vi "motor control 4.vi"(0 "Fine":u16, 1 "proportional gain (Kc)":dbl, 2 "Manual control":dbl, 3 "reinitialize? (F)":bool, 4 "derivative time (Td, min)":dbl, 5 "error in (no error)":errorcluster, 6 "integral time (Ti, min)":dbl, 7 "cycle\"i\"":i32, 8 "velocità desiderata":dbl, 9 "Stoppa ciclo":bool, 10 "offset":dbl, 11 "auto? (T)":bool=TRUE, 12 "delta t":u32) -> (14 "pwm out":dbl, 15 "Boolean":bool, 19 "error out":errorcluster)   [LabVIEW 2017]
uses:
  <vilib>/functionblocks/Control/PID/PID.vi
  <vilib>/functionblocks/FB Core/FB Core.xnode
  <vilib>/functionblocks/FB Property/FB Overlay DBL.ctl
  <vilib>/functionblocks/NI_FunctionBlock Libraries.lvlib
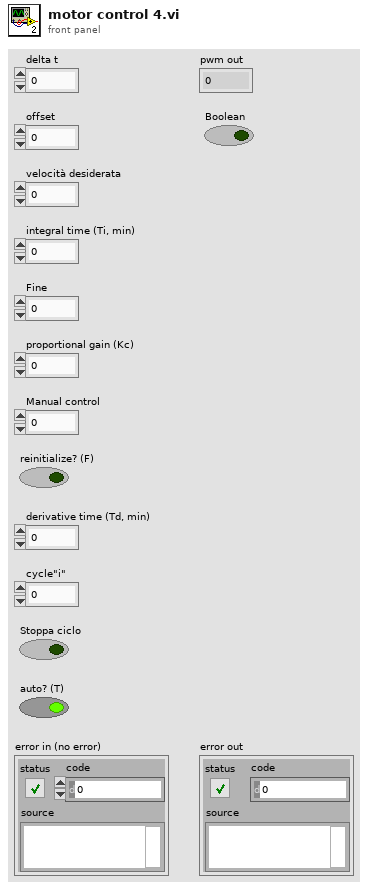
[diagram p1: front panel]
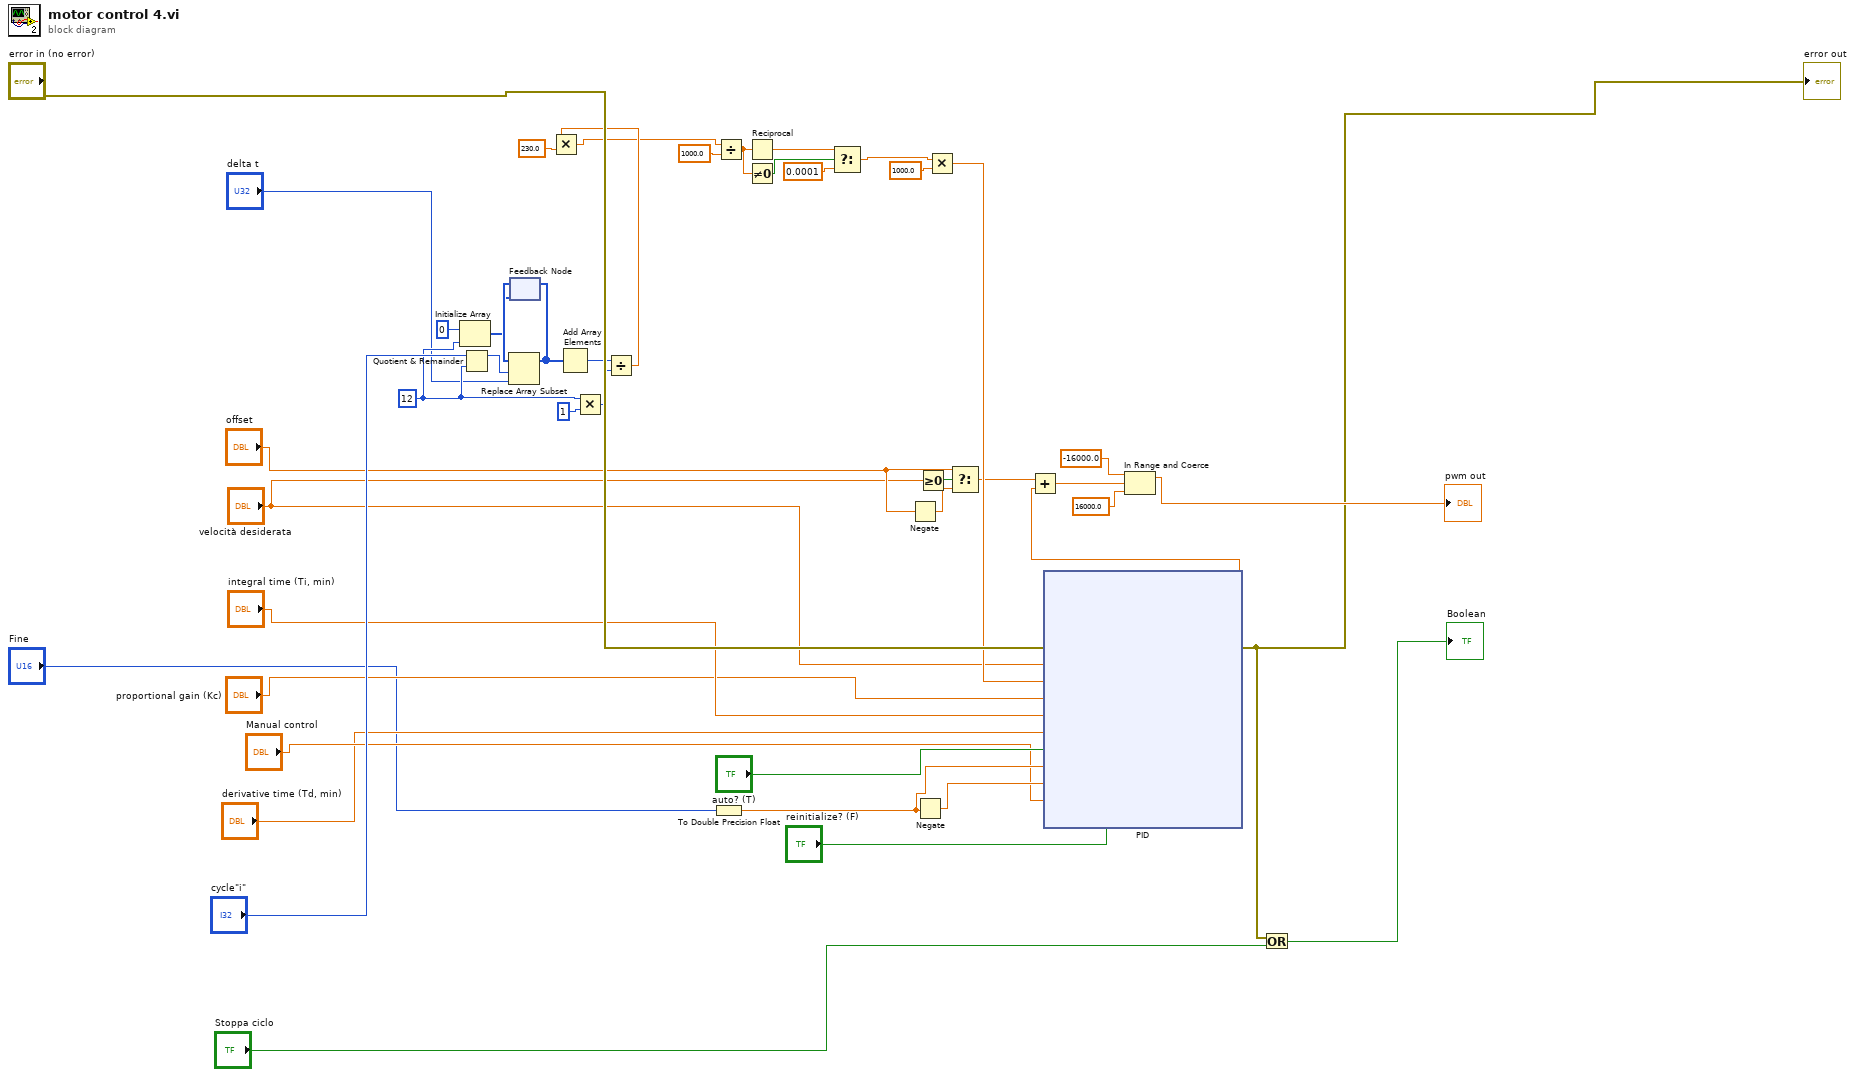
[diagram p0: block diagram]
diagram:
  w39 = 12 ("dimension size")
  n1 = Initialize Array(0, w39) -> (w40:i32[])
  n2 = Quotient & Remainder(x="cycle\"i\"", y=w39) -> (x-y*floor(x/y)=w32:i32)  [unwired: 1 out]
  n3 = feedback #1(w40) -> (w42:i32[])
  n4 = Replace Array Subset(array=w42, new element="delta t", index=w32) -> (w41:i32[])
  n5 = feedback-in #1(w41) -> ()
  n6 = Add Array Elements(numeric array=w41) -> (sum=w21:i32)
  n7 = Multiply(x=w39, y=1) -> (x*y=w34:i32)
  n8 = Divide(x=w21, y=w34) -> (x/y=w22:dbl)
  n9 = Multiply(x=w22, y=230.0) -> (x*y=w16:dbl)
  n10 = To Double Precision Float(number="Fine") -> (double precision float=w31:dbl)
  n11 = Divide(x=w16, y=1000.0) -> (x/y=w18:dbl)
  n12 = Reciprocal(x=w18) -> (1/x=w12:dbl)
  n13 = Not Equal To 0?(x=w18) -> (x != 0?=w13:bool)
  n14 = Select(t=w12, s=w13, f=0.0001) -> (s? t:f=w19:dbl)
  n15 = Negate(x="offset") -> (-x=w24:dbl)
  n16 = Negate(x=w31) -> (-x=w30:dbl)
  n17 = Greater Or Equal To 0?(x="velocità desiderata") -> (x >= 0?=w25:bool)
  n18 = Multiply(x=w19, y=1000.0) -> (x*y=w37:dbl)
  n19 = Select(t="offset", s=w25, f=w24) -> (s? t:f=w23:dbl)
  n20 = xnode "PID"("error in"="error in (no error)", "setpoint"="velocità desiderata", "process variable"=w37, "proportional gain (Kc)"="proportional gain (Kc)", "integral time (Ti, min)"="integral time (Ti, min)", "derivative time (Td, min)"="derivative time (Td, min)", "auto? (T)"="auto? (T)", "output high"=w31, "output low"=w30, "manual control"="Manual control", "reinitialize? (F)"="reinitialize? (F)") -> ("error out"=w2:errorcluster, "output"=w36:dbl)
  "error out" <- w2
  n21 = Add(x=w23, y=w36) -> (x+y=w28:dbl)
  n22 = In Range and Coerce(upper limit=-16000.0, x=w28, lower limit=16000.0) -> (coerced(x)=→"pwm out":dbl)  [unwired: 1 out]
  n23 = Or(x=w2, y="Stoppa ciclo") -> (x .or. y?=→"Boolean":bool)
